vi "User Interface.vi"(8 "error in":errorcluster, 11 "Inset In":refnum<class "Inset.lvclass">) -> (0 "error out":errorcluster, 3 "Inset Out":refnum<class "Inset.lvclass">)   [LabVIEW 2019, in "Inset.lvclass"]
uses:
  Inset.lvclass
  BigMAQ/BigMAQ.lvclass
  Parse/ParseXML/Image.ctl
  Parse/ParseXML/ParseSVG.lvclass
  Parse/EditSVG/EditSVG.lvclass
  <vilib>/LabVIEW Open Source Project/OpenURI/openURI.lvlib
  <vilib>/LabVIEW Open Source Project/Data Manipulation/Scalar/OpenScalar.lvlib
panel:
  in  "Apply":bool
  in  "Cancel":bool
  out "SVG File":path caption="Path"
  in  "Inset Page":u32 caption="Numeric" max=3
  in  "Inset Data Range":cluster{sgl, sgl}(slide)={100.0, 0.0} scale=0.0..100.0
  in  "Inset Image":path caption="Path"
  in  "Background Page":u32 caption="Numeric" max=3
  in  "Background Data Range":cluster{sgl, sgl}(slide)={100.0, 0.0} scale=0.0..100.0
  out "Background Image":path caption="Path"
  in  "Inset Collapse":bool
  out "INST Render":T1(plugin-control)
  in  "Background Collapse":bool
  out "BGND Render":T1(plugin-control)
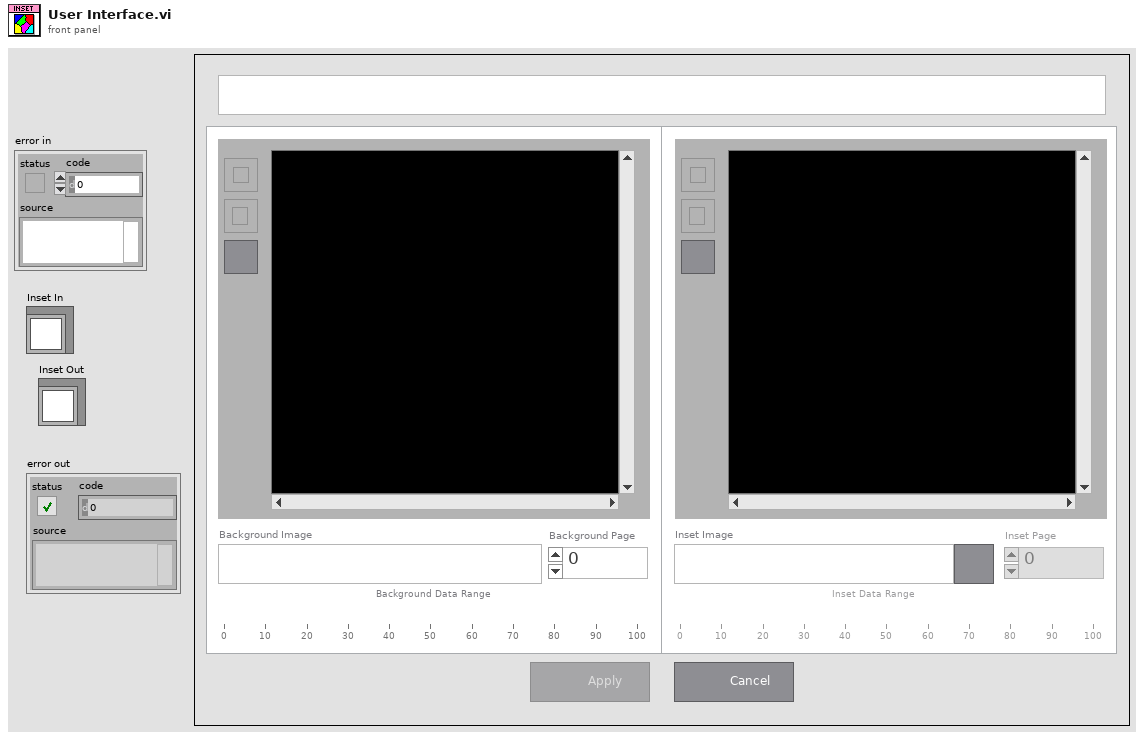
[diagram p1: front panel]
types:
  T1 = typedef "IMAQ Image.ctl" = refnum<image>
  T2 = enum32{"Invalid", "Standard", "Closed", "Hidden", "Minimized", "Maximized"}
  T3 = enum32{"invalid app kind", "Development System", "Run Time System", "Student Edition", "Embedded LabVIEW", "Evaluation", "Custom"}
  T4 = enum8{"Enabled", "Disabled", "Disabled and Grayed Out"}
  T5 = typedef "ParseSVG.lvclass/Image.ctl" = cluster{"x":string, "y":string, "width":string, "height":string, "xlink:href":string, "id":string, "transform":string}
  T6 = cluster{"Core":cluster{"Current VI Reference":refnum<vi>, "Close Panel on Exit?":bool}, "BGND Data":cluster{"YOffset":dbl, "XOffset":dbl, "ScanSize":dbl}, "INST Data":cluster{"YOffset":dbl, "XOffset":dbl, "ScanSize":dbl}, "SVG Image Data":T5, "Exists?":bool, "Existing id":string}
  T7 = cluster{"YOffset":dbl, "XOffset":dbl, "ScanSize":dbl}
  T8 = cluster{"Current VI Reference":refnum<vi>, "Close Panel on Exit?":bool}
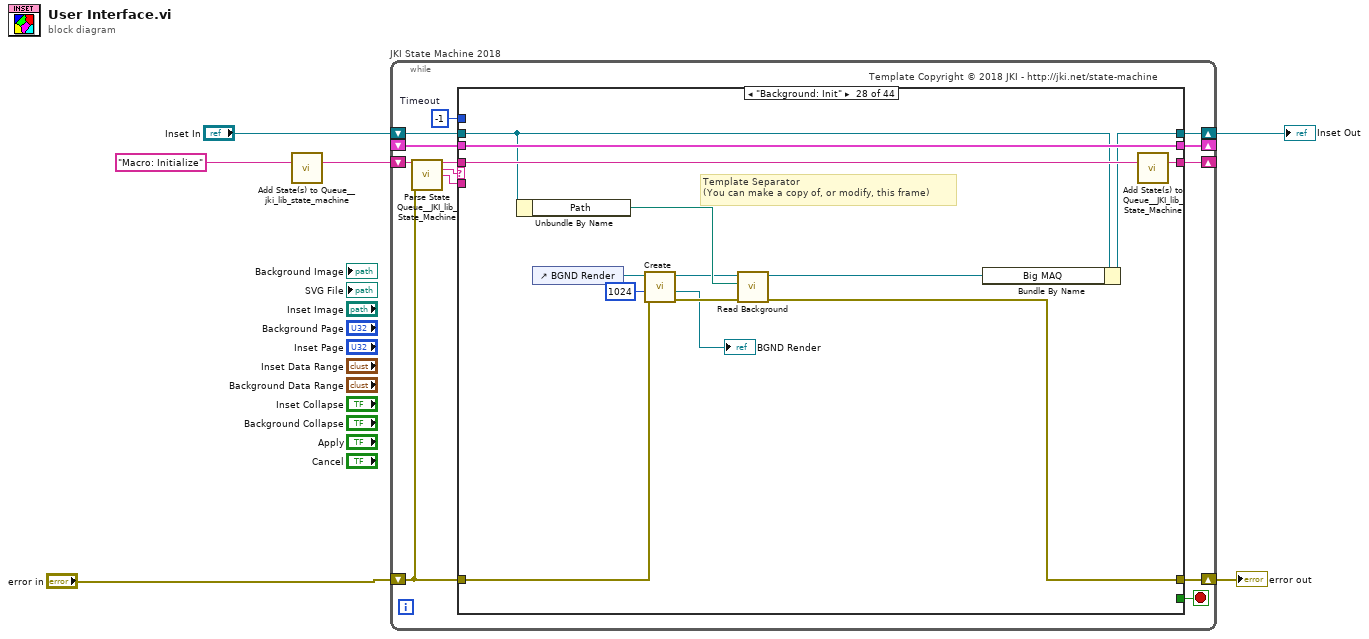
[diagram p0: block diagram]
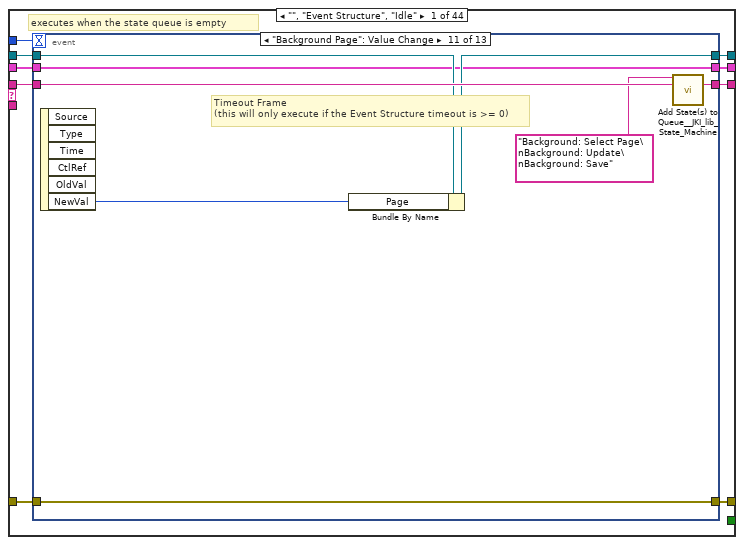
[diagram p2: hidden frame]
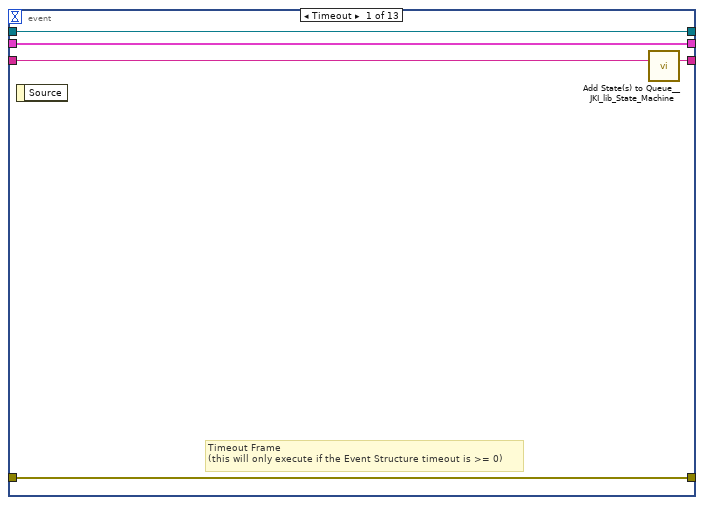
[diagram p3: hidden frame]
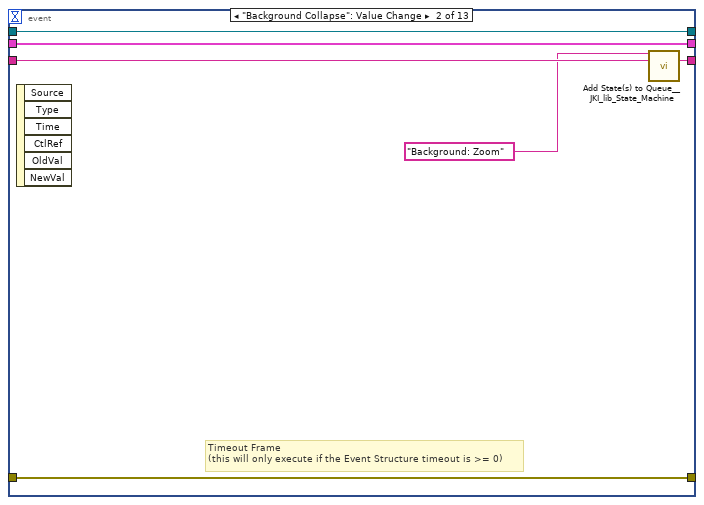
[diagram p4: hidden frame]
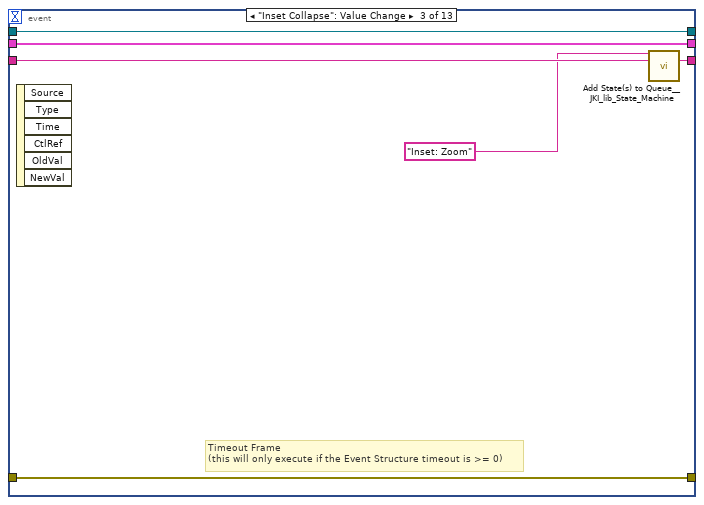
[diagram p5: hidden frame]
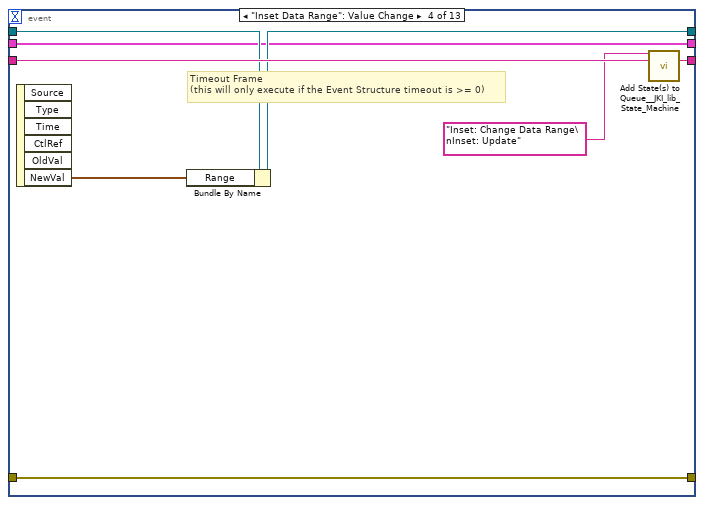
[diagram p6: hidden frame]
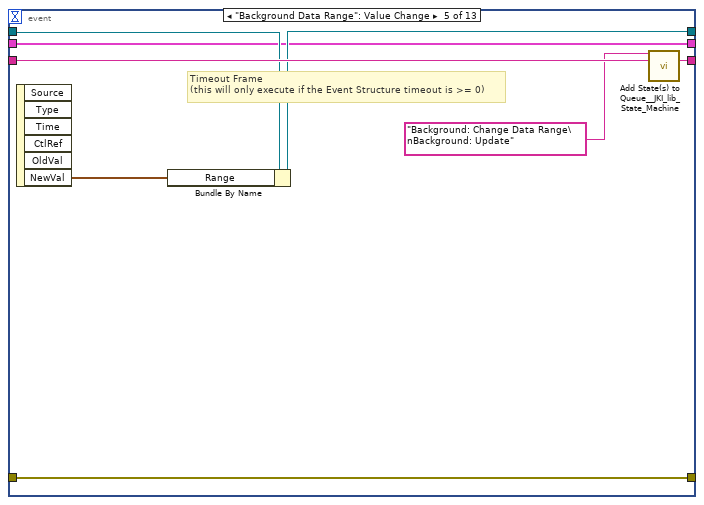
[diagram p7: hidden frame]
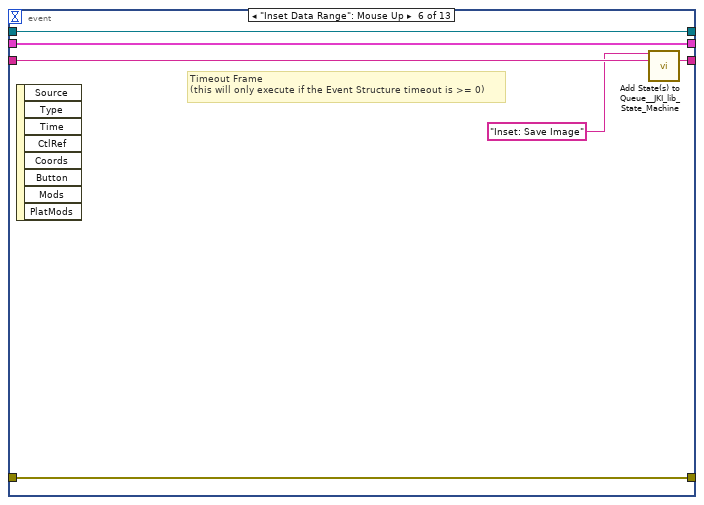
[diagram p8: hidden frame]
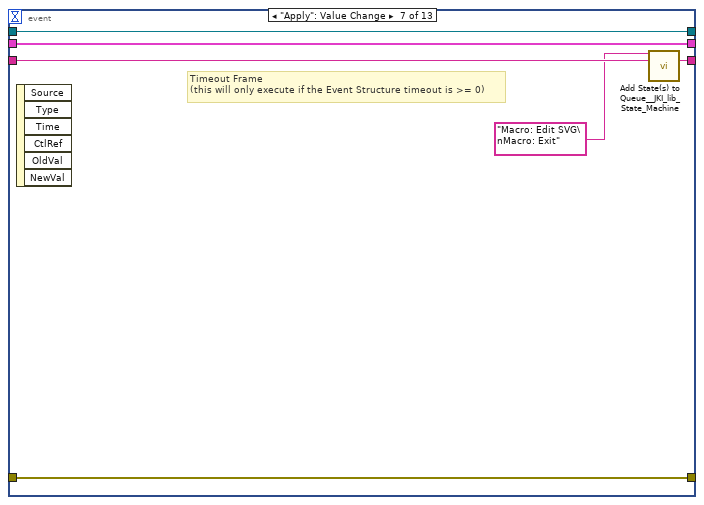
[diagram p9: hidden frame]
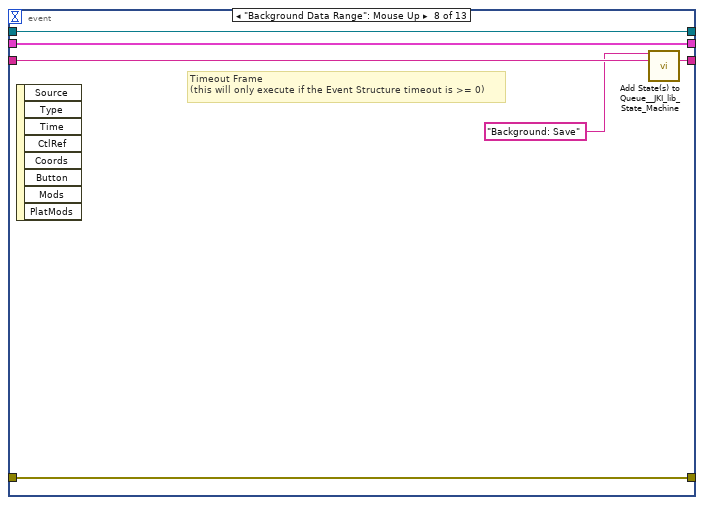
[diagram p10: hidden frame]
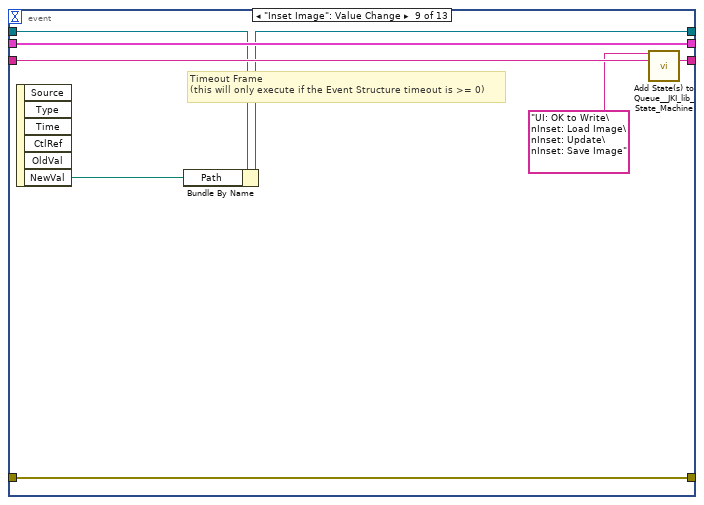
[diagram p11: hidden frame]
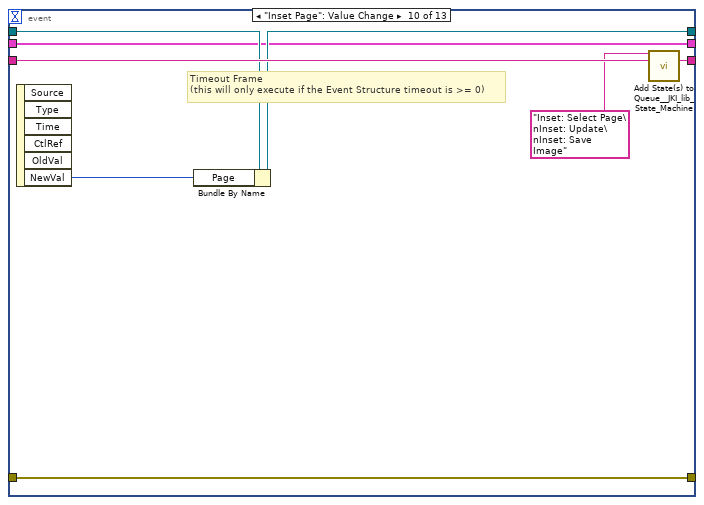
[diagram p12: hidden frame]
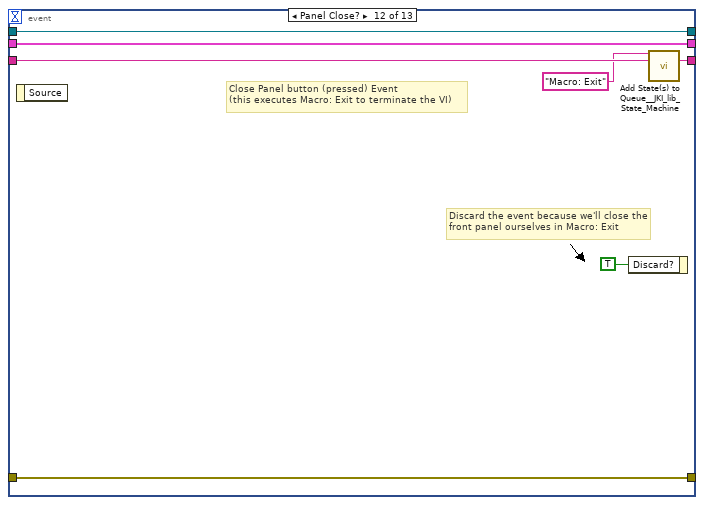
[diagram p13: hidden frame]
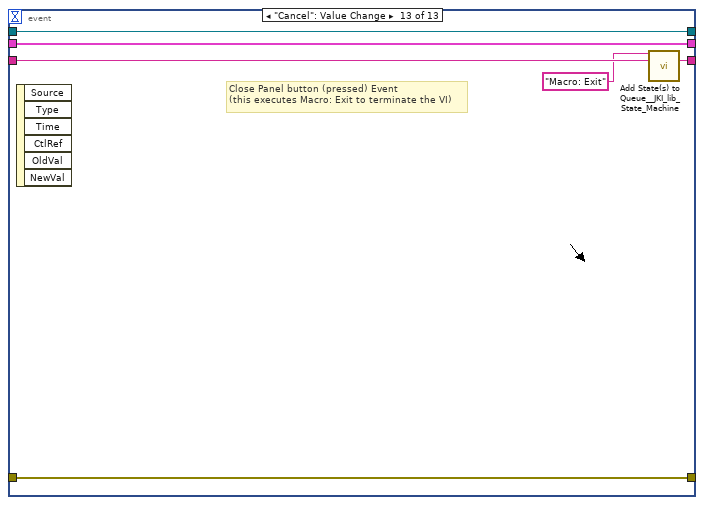
[diagram p14: hidden frame]
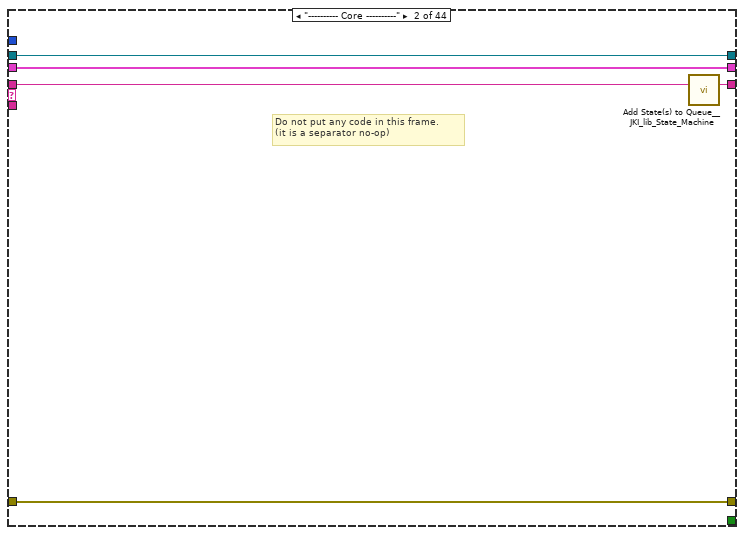
[diagram p15: hidden frame]
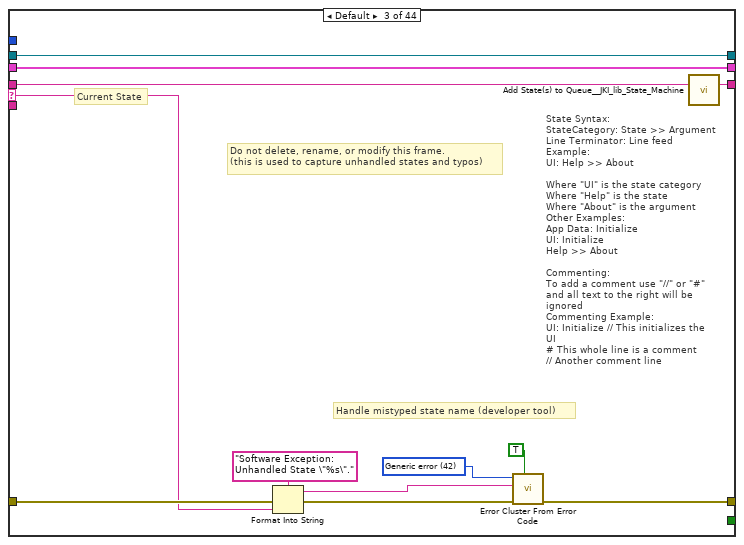
[diagram p16: hidden frame]
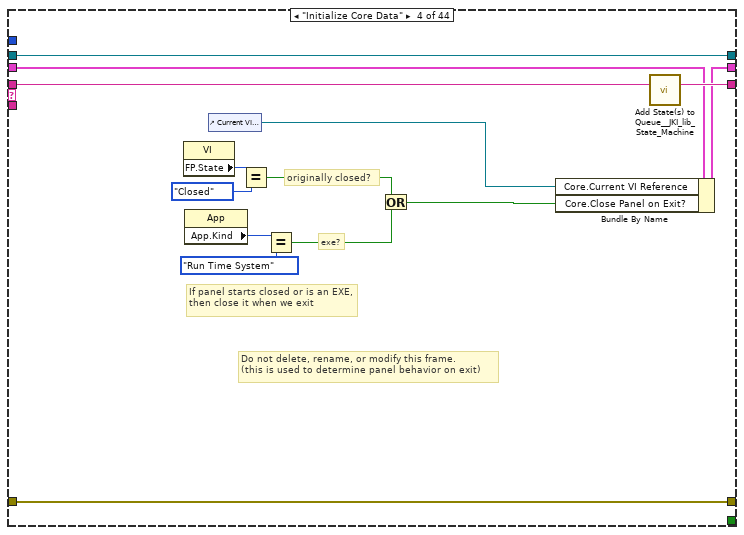
[diagram p17: hidden frame]
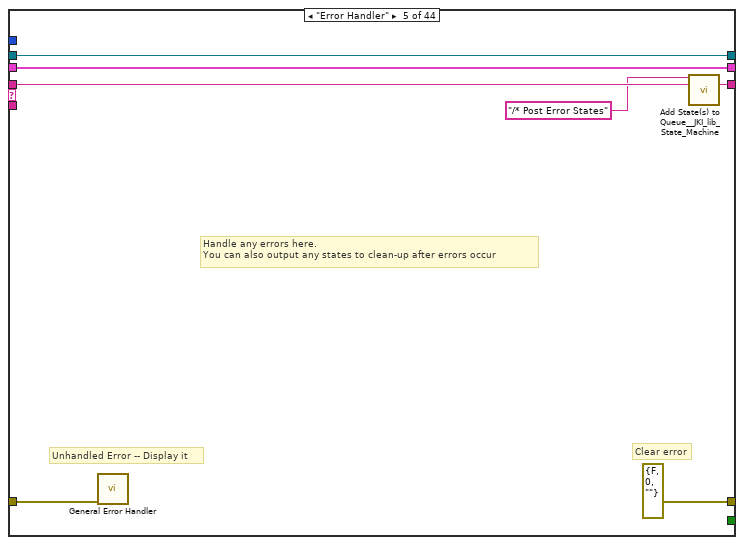
[diagram p18: hidden frame]
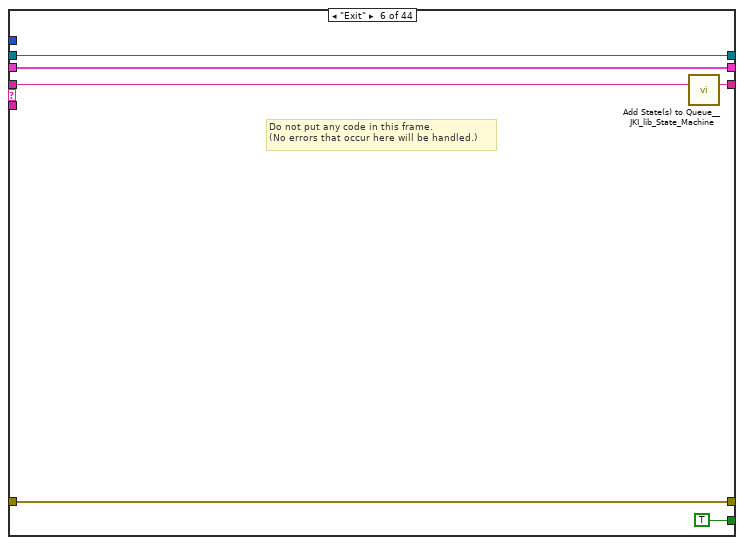
[diagram p19: hidden frame]
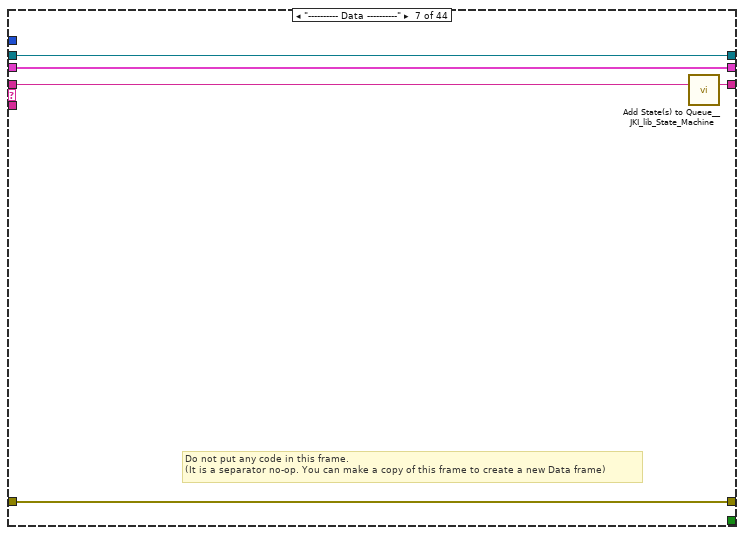
[diagram p20: hidden frame]
diagram:
  n1 = call <vilib>:"Add State(s) to Queue__jki_lib_state_machine.vi"("State(s) in (\"\")"="Macro: Initialize") -> ("States Out"=w6:string)  [unwired: 14 in]
  n2 = while "JKI State Machine 2018" {
    shift-right: [w12] -> _
    shift-left: _ -> [w11]
    shift-right: [w15] -> w4
    shift-left: "error in" -> [w9]
    shift-right: [w14] -> _
    shift-left: w6 -> [w16]
    shift-right: [w7] -> w1
    shift-left: "Inset In" -> [w8]
    stop <- w13 stop-if-true
    w10 = -1  # Timeout
    # "Template Copyright © 2018 JKI - http://jki.net/state-machine"
    n3 = call <vilib>:"Parse State Queue__JKI_lib_State_Machine.vi"("State Queue"=w16, "Error In (no error)"=w9) -> ("Remaining States"=w18:string, "Current State"=w19:string, "Arguments"=w17:string)  [unwired: 11 in]
    n4 = case shown="\"Background: Init\"" w19 {
      selector: w19 -> [_ _ w123 _ _ _ _ _ _ _ _ _ _ _ _ _ _ _ _ _ _ _ _ _ _ _ _ _ _ _ _ _ _ _ _ _ _ _ _ _ _ _ _ _]
      tunnel: w18 -> [w28 w121 w127 w147 w154 w160 w165 w176 w183 w188 w204 w219 w226 w238 w308 w314 w320 w331 w342 w347 w361 w383 w392 w404 w417 w442 w449 w463 w479 w493 w504 w515 w524 w533 w542 w549 w558 w567 w587 w598 w612 w624 w636 w645]
      tunnel: w17 -> [_ _ _ _ _ _ _ _ _ _ _ _ w221 w232 _ _ _ _ _ _ _ _ _ _ _ _ _ _ _ _ _ _ _ _ _ _ _ _ _ _ _ _ _ _]
      tunnel: w11 -> [w26 w118 w125 w140 w151 w158 w162 _ w178 w185 w202 w207 w224 w234 w305 w311 w317 w327 w339 w344 w349 w370 w385 w393 w405 w426 w446 w461 w477 w484 w498 w509 w520 w531 w536 w545 w556 w561 w584 w590 w599 w615 w629 w637]
      tunnel: [w25 w119 w129 w144 errorcluster {"status"=FALSE, "code"=0, "source"=""} ("error out") w157 w163 w173 w179 w186 w190 w209 w222 w235 w306 w312 w318 w329 w340 w345 w357 w381 w390 w396 w410 w440 w447 w452 w468 w486 w500 w513 w522 w526 w538 w547 w551 w563 w575 w594 w608 w620 w631 w641] -> w15
      tunnel: w9 -> [w24 w119 w128 w144 w150 w157 w163 w173 w180 w186 w196 w208 w223 w236 w306 w312 w318 w329 w340 w345 w354 w381 w390 w395 w409 w440 w447 w459 w475 w485 w499 w512 w521 w525 w537 w547 w550 w562 w583 w593 w607 w619 w630 w640]
      tunnel: [w27 w120 w126 w146 w153 w159 w164 w175 w182 w187 w203 w218 w225 w237 w307 w313 w319 w330 w341 w346 w360 w382 w391 w403 w416 w441 w448 w462 w478 w492 w503 w514 w523 w532 w541 w548 w557 w566 w586 w597 w611 w623 w635 w644] -> w14
      tunnel: [_ _ _ _ _ TRUE _ _ _ _ _ _ _ _ _ _ _ _ _ _ _ _ _ _ _ _ _ _ _ _ _ _ _ _ _ _ _ _ _ _ _ _ _ _] -> w13
      tunnel: [w23 w118 w125 w145 w151 w158 w162 w174 w178 w185 w202 w207 w224 w234 w305 w311 w317 w327 w339 w344 w349 w371 w385 w393 w405 w426 w446 w461 w476 w484 w498 w509 w520 w531 w536 w545 w556 w561 w585 w590 w599 w615 w629 w637] -> w12
      tunnel: w10 -> [w22 _ _ _ _ _ _ _ _ _ _ _ _ _ _ _ _ _ _ _ _ _ _ _ _ _ _ _ _ _ _ _ _ _ _ _ _ _ _ _ _ _ _ _]
      tunnel: w8 -> [w21 w117 w122 w134 w148 w155 w161 w171 w177 w184 w201 w217 w220 w231 w304 w309 w315 w321 w332 w343 w352 w376 w388 w394 w406 w424 w444 w456 w464 w482 w494 w505 w516 w529 w534 w543 w554 w559 w570 w591 w600 w613 w627 w638]
      tunnel: [w20 w117 w122 w134 w148 w155 w161 w171 w177 w184 w201 w217 w220 w231 w304 w309 w315 w321 w332 w343 w353 w377 w386 w394 w407 w425 w445 w460 w465 w483 w495 w506 w517 w530 w535 w544 w555 w560 w571 w592 w601 w614 w628 w639] -> w7
      frame "", "Event Structure", "Idle" {
        # "executes when the state queue is empty"
        n5 = event shown="[10] \"Background Page\": Value Change" {
          selector: _ -> [_ _ _ _ _ _ _ _ _ _ _ _ _]
          dyn-events: _ -> [_ _ _ _ _ _ _ _ _ _ _ _ _]
          timeout: w22 -> [_ _ _ _ _ _ _ _ _ _ _ _ _]
          tunnel: w28 -> [w33 w39 w45 w53 w61 w67 w73 w79 w87 w95 w103 w110 w116]
          tunnel: [w32 w38 w44 w52 w60 w66 w72 w78 w86 w94 w102 w109 w115] -> w27
          tunnel: w26 -> [w30 w36 w42 w46 w55 w63 w69 w75 w82 w88 w96 w107 w113]
          tunnel: [w31 w37 w43 w51 w59 w65 w71 w77 w85 w93 w101 w108 w114] -> w25
          tunnel: w24 -> [w31 w37 w43 w51 w59 w65 w71 w77 w85 w93 w101 w108 w114]
          tunnel: [w30 w36 w42 w46 w55 w63 w69 w75 w82 w88 w96 w107 w113] -> w23
          tunnel: w21 -> [w29 w35 w41 w47 w56 w62 w68 w74 w80 w89 w98 w104 w111]
          tunnel: [w29 w35 w41 w48 w57 w62 w68 w74 w81 w90 w99 w104 w111] -> w20
          event Timeout {
            # "Timeout Frame\n(this will only execute if the Event Structure timeout is >= 0)"
            n6 = event-data() -> ()  [unwired: 1 in, 1 out]
            n7 = call <vilib>:"Add State(s) to Queue__JKI_lib_State_Machine.vi"("State(s) in (\"\")"=w33) -> ("States Out"=w32:string)  [unwired: 14 in]
          }
          event "Background Collapse": Value Change {
            # "Timeout Frame\n(this will only execute if the Event Structure timeout is >= 0)"
            n8 = event-data() -> ()  [unwired: 1 in, 6 out]
            n9 = call <vilib>:"Add State(s) to Queue__JKI_lib_State_Machine.vi"("State(s) in Front (\"\")"="Background: Zoom", "State(s) in (\"\")"=w39) -> ("States Out"=w38:string)  [unwired: 13 in]
          }
          event "Inset Collapse": Value Change {
            # "Timeout Frame\n(this will only execute if the Event Structure timeout is >= 0)"
            n10 = event-data() -> ()  [unwired: 1 in, 6 out]
            n11 = call <vilib>:"Add State(s) to Queue__JKI_lib_State_Machine.vi"("State(s) in Front (\"\")"="Inset: Zoom", "State(s) in (\"\")"=w45) -> ("States Out"=w44:string)  [unwired: 13 in]
          }
          event "Inset Data Range": Value Change {
            # "Timeout Frame\n(this will only execute if the Event Structure timeout is >= 0)"
            n12 = event-data() -> ("NewVal"=w49:cluster{sgl, sgl})  [unwired: 1 in, 5 out]
            n13 = Bundle By Name(cluster=w47, "Range"=w49) -> (w48:refnum<class "Inset.lvclass">)
            n14 = call <vilib>:"Add State(s) to Queue__JKI_lib_State_Machine.vi"("State(s) in Front (\"\")"="Inset: Change Data Range\nInset: Update" ("State(s) in Front (\"\")"), "State(s) in (\"\")"=w53) -> ("States Out"=w52:string)  [unwired: 13 in]
          }
          event "Background Data Range": Value Change {
            # "Timeout Frame\n(this will only execute if the Event Structure timeout is >= 0)"
            n15 = event-data() -> ("NewVal"=w54:cluster{sgl, sgl})  [unwired: 1 in, 5 out]
            n16 = Bundle By Name(cluster=w56, "Range"=w54) -> (w57:refnum<class "Inset.lvclass">)
            n17 = call <vilib>:"Add State(s) to Queue__JKI_lib_State_Machine.vi"("State(s) in Front (\"\")"="Background: Change Data Range\nBackground: Update" ("State(s) in Front (\"\")"), "State(s) in (\"\")"=w61) -> ("States Out"=w60:string)  [unwired: 13 in]
          }
          event "Inset Data Range": Mouse Up {
            # "Timeout Frame\n(this will only execute if the Event Structure timeout is >= 0)"
            n18 = event-data() -> ()  [unwired: 1 in, 8 out]
            n19 = call <vilib>:"Add State(s) to Queue__JKI_lib_State_Machine.vi"("State(s) in Front (\"\")"="Inset: Save Image" ("State(s) in Front (\"\")"), "State(s) in (\"\")"=w67) -> ("States Out"=w66:string)  [unwired: 13 in]
          }
          event "Apply": Value Change {
            # "Timeout Frame\n(this will only execute if the Event Structure timeout is >= 0)"
            n20 = event-data() -> ()  [unwired: 1 in, 6 out]
            n21 = call <vilib>:"Add State(s) to Queue__JKI_lib_State_Machine.vi"("State(s) in Front (\"\")"="Macro: Edit SVG\nMacro: Exit" ("State(s) in Front (\"\")"), "State(s) in (\"\")"=w73) -> ("States Out"=w72:string)  [unwired: 13 in]
          }
          event "Background Data Range": Mouse Up {
            # "Timeout Frame\n(this will only execute if the Event Structure timeout is >= 0)"
            n22 = event-data() -> ()  [unwired: 1 in, 8 out]
            n23 = call <vilib>:"Add State(s) to Queue__JKI_lib_State_Machine.vi"("State(s) in Front (\"\")"="Background: Save" ("State(s) in Front (\"\")"), "State(s) in (\"\")"=w79) -> ("States Out"=w78:string)  [unwired: 13 in]
          }
          event "Inset Image": Value Change {
            # "Timeout Frame\n(this will only execute if the Event Structure timeout is >= 0)"
            n24 = event-data() -> ("NewVal"=w83:path)  [unwired: 1 in, 5 out]
            n25 = Bundle By Name(cluster=w80, "Path"=w83) -> (w81:refnum<class "Inset.lvclass">)
            n26 = call <vilib>:"Add State(s) to Queue__JKI_lib_State_Machine.vi"("State(s) in Front (\"\")"="UI: OK to Write\nInset: Load Image\nInset: Update\nInset: Save Image" ("State(s) in Front (\"\")"), "State(s) in (\"\")"=w87) -> ("States Out"=w86:string)  [unwired: 13 in]
          }
          event "Inset Page": Value Change {
            # "Timeout Frame\n(this will only execute if the Event Structure timeout is >= 0)"
            n27 = event-data() -> ("NewVal"=w91:u32)  [unwired: 1 in, 5 out]
            n28 = Bundle By Name(cluster=w89, "Page"=w91) -> (w90:refnum<class "Inset.lvclass">)
            n29 = call <vilib>:"Add State(s) to Queue__JKI_lib_State_Machine.vi"("State(s) in Front (\"\")"="Inset: Select Page\nInset: Update\nInset: Save Image" ("State(s) in Front (\"\")"), "State(s) in (\"\")"=w95) -> ("States Out"=w94:string)  [unwired: 13 in]
          }
          event "Background Page": Value Change {
            # "Timeout Frame\n(this will only execute if the Event Structure timeout is >= 0)"
            n30 = event-data() -> ("NewVal"=w97:u32)  [unwired: 1 in, 5 out]
            n31 = Bundle By Name(cluster=w98, "Page"=w97) -> (w99:refnum<class "Inset.lvclass">)
            n32 = call <vilib>:"Add State(s) to Queue__JKI_lib_State_Machine.vi"("State(s) in Front (\"\")"="Background: Select Page\nBackground: Update\nBackground: Save" ("State(s) in Front (\"\")"), "State(s) in (\"\")"=w103) -> ("States Out"=w102:string)  [unwired: 13 in]
          }
          event Panel Close? {
            # "Discard the event because we'll close the front panel ourselves in Macro: Exit"
            # "Close Panel button (pressed) Event\n(this executes Macro: Exit to terminate the VI)"
            n33 = event-data() -> ()  [unwired: 1 in, 1 out]
            n34 = event-data("Discard?"=TRUE) -> ()  [unwired: 1 in, 1 out]
            n35 = call <vilib>:"Add State(s) to Queue__JKI_lib_State_Machine.vi"("State(s) in Front (\"\")"="Macro: Exit", "State(s) in (\"\")"=w110) -> ("States Out"=w109:string)  [unwired: 13 in]
          }
          event "Cancel": Value Change {
            # "Close Panel button (pressed) Event\n(this executes Macro: Exit to terminate the VI)"
            n36 = event-data() -> ()  [unwired: 1 in, 6 out]
            n37 = call <vilib>:"Add State(s) to Queue__JKI_lib_State_Machine.vi"("State(s) in Front (\"\")"="Macro: Exit", "State(s) in (\"\")"=w116) -> ("States Out"=w115:string)  [unwired: 13 in]
          }
        }
      }
      frame "---------- Core ----------" {
        # "Do not put any code in this frame.\n(it is a separator no-op)"
        n38 = call <vilib>:"Add State(s) to Queue__JKI_lib_State_Machine.vi"("State(s) in (\"\")"=w121) -> ("States Out"=w120:string)  [unwired: 14 in]
      }
      frame Default {
        w132 = 42 items=["No error", "Argument error", "Memory is full", "Out of zone", "End of file", "File already open", "Generic file I/O error", "File not found", "File permission error", "Disk is full", "Duplicate path", "Too many files open", "System feature not enabled", "Resource file not found", "Cannot add resource", "Resource not found", "Image not found", "Image memory error", "Pen does not exist", "Config type invalid", "Config token not found", "Config parse error", "Config memory error", "Bad external code format", "Bad external code offset", "External code not present", "Null window", "Destroy window error", "Null menu", "Print aborted", "Bad print record", "Print driver error", "Windows error during printing", "Memory error during printing", "Print dialog error", "Generic print error", "Invalid device refnum", "Device not found", "Device parameter error", "Device unit error", "Cannot open device", "Device call aborted", "Generic error", "Cancelled by user", "Object ID too low", "Object ID too high", "Object not in heap", "Unknown heap", "Unknown object (invalid DefProc)", "Unknown object (DefProc not in table)", "Message out of range", "Invalid (null) method", "Unknown message", "Manager call not supported", "Bad address", "Network operation in progress", "Network operation timed out", "Connection is busy", "Network attribute not supported", "Network error", "Address in use", "System out of memory", "Connection aborted", "Connection refused", "Not connected", "Already connected", "Connection closed", "Initialization error (interapplication manager)", "Bad occurrence", "Wait on unbound occurrence handler", "Occurrence queue overflow", "Datalog type conflict", "Unused", "Unrecognized type (interapplication manager)", "Memory corrupt", "Failed to make temporary DLL", "Old CIN version", "Drag socket not found", "Failed to load drop-object", "Failed to register OLE object", "Failed to release OLE object", "Format specifier type mismatch", "Unknown format specifier", "Too few format specifiers", "Too many format specifiers", "Scan failed", "Newer CIN version", "Error converting to variant", "Runtime menu error", "Password tampered", "Variant attribute not found", "Incompatible variant data type", "Event data is not available", "Event Store is not present", "Occurrence is not found", "Event Queue is not created", "Event info is not available", "Refnum passed is NULL", "Error retrieving Class GUID", "Error retrieving CoClass GUID", "Error retrieving TypeLib GUID.", "Bad built application magic bytes.", "Specific driver is different from the specific driver associated with the Logical Name.", "There is no session opened to the class driver.", "Max Error", "MAX - Error with config objects", "MAX - Error loading configuration", "MAX - Group not supported"]
        # "State Syntax:\nStateCategory: State >> Argument\nLine Terminator: Line feed\nExample:\nUI: Help >> About\n\nWhere \"UI\" is the state category\nWhere \"Help\" is the state\nWhere \"About\" is the argument\nOther Examples:\nApp Data: Initialize\nUI: Initialize\nHelp >> About\n\nCommenting:\nTo add a comment use \"//\" or \"#\" and all text to the right will be ignored\nCommenting Example:\nUI: Initialize // This initializes the UI\n# This whole line is a comment\n// Another comment line"
        # "Current State"
        # "Do not delete, rename, or modify this frame.\n(this is used to capture unhandled states and typos)"
        # "Handle mistyped state name (developer tool)"
        n39 = Format Into String(format string="Software Exception: Unhandled State \"%s\"." ("message"), error in=w128, w123) -> (resulting string=w131:string, error out=w130:errorcluster)  [unwired: 1 in]
        n40 = call <vilib>:"Error Cluster From Error Code.vi"("show call chain? (False)"=TRUE, "error in (no error)"=w130, "error message (\"\")"=w131, "error code (0)"=w132) -> ("error out"=w129:errorcluster)  [unwired: 5 in]
        n41 = call <vilib>:"Add State(s) to Queue__JKI_lib_State_Machine.vi"("State(s) in (\"\")"=w127) -> ("States Out"=w126:string)  [unwired: 14 in]
      }
      frame "Initialize Core Data" {
        # "Do not delete, rename, or modify this frame.\n(this is used to determine panel behavior on exit)"
        # "originally closed?"
        # "exe?"
        # "If panel starts closed or is an EXE, then close it when we exit"
        n42 = property class="VI"() -> ("FP.State"=w137:T2)  [unwired: 2 in, 2 out]
        n43 = property class="App"() -> ("App.Kind"=w143:T3)  [unwired: 2 in, 2 out]
        n44 = control-ref of="Current VI Reference"() -> (w138:refnum<vi>)
        n45 = Equal?(x=w137, y=T2."Closed" ("Front Panel Window:State")) -> (x = y?=w135:bool)
        n46 = Equal?(x=w143, y=T3."Run Time System" ("Application:Kind")) -> (x = y?=w141:bool)
        n47 = Or(x=w135, y=w141) -> (x .or. y?=w139:bool)
        n48 = Bundle By Name(cluster=w140, "Core.Current VI Reference"=w138, "Core.Close Panel on Exit?"=w139) -> (w145:T6)
        n49 = call <vilib>:"Add State(s) to Queue__JKI_lib_State_Machine.vi"("State(s) in (\"\")"=w147) -> ("States Out"=w146:string)  [unwired: 14 in]
      }
      frame "Error Handler" {
        # "Unhandled Error -- Display it"
        # "Handle any errors here.\nYou can also output any states to clean-up after errors occur"
        # "Clear error"
        n50 = call <vilib>:"General Error Handler.vi"("error in (no error)"=w150) -> ()  [unwired: 10 in, 5 out]
        n51 = call <vilib>:"Add State(s) to Queue__JKI_lib_State_Machine.vi"("State(s) in Front (\"\")"="/* Post Error States", "State(s) in (\"\")"=w154) -> ("States Out"=w153:string)  [unwired: 13 in]
      }
      frame "Exit" {
        # "Do not put any code in this frame.\n(No errors that occur here will be handled.)"
        n52 = call <vilib>:"Add State(s) to Queue__JKI_lib_State_Machine.vi"("State(s) in (\"\")"=w160) -> ("States Out"=w159:string)  [unwired: 14 in]
      }
      frame "---------- Data ----------" {
        # "Do not put any code in this frame.\n(It is a separator no-op. You can make a copy of this frame to create a new Data frame)"
        n53 = call <vilib>:"Add State(s) to Queue__JKI_lib_State_Machine.vi"("State(s) in (\"\")"=w165) -> ("States Out"=w164:string)  [unwired: 14 in]
      }
      frame "Data: Initialize" {
        w166 = ""  # Existing id
        w167 = FALSE  # Exists?
        w168 = T5 {"x"="", "y"="", "width"="", "height"="", "xlink:href"="", "id"="", "transform"=""}  # SVG Image Data
        w169 = T7 {"YOffset"=0.0, "XOffset"=0.0, "ScanSize"=0.0}  # INST Data
        w170 = T7 {"YOffset"=0.0, "XOffset"=0.0, "ScanSize"=0.0}  # BGND Data
        w172 = T8 {"Current VI Reference"=refnum, "Close Panel on Exit?"=FALSE}  # Core
        # "do not delete - used by framework"
        # "Data names and types of shift register data are defined by this bundle."
        # "Initialize the shift-register data, here.\n(data names are defined by what you wire into the bundle function)"
        n54 = Bundle("Core"=w172, "BGND Data"=w170, "INST Data"=w169, "SVG Image Data"=w168, "Exists?"=w167, "Existing id"=w166) -> (w174:T6)  [unwired: 1 in]
        n55 = call <vilib>:"Add State(s) to Queue__JKI_lib_State_Machine.vi"("State(s) in (\"\")"=w176) -> ("States Out"=w175:string)  [unwired: 14 in]
      }
      frame "Data: Cleanup" {
        # "Cleanup any data and references, here.\n(this is called automatically, by the Macro: Exit)"
        n56 = Unbundle By Name(w178) -> ("Core.Current VI Reference"=w181:refnum<vi>)
        n57 = Close Reference(reference=w181, error in (no error)=w180) -> (error out=w179:errorcluster)
        n58 = call <vilib>:"Add State(s) to Queue__JKI_lib_State_Machine.vi"("State(s) in (\"\")"=w183) -> ("States Out"=w182:string)  [unwired: 14 in]
      }
      frame "---------- UI ----------" {
        # "Do not put any code in this frame.\n(It is a separator no-op. You can make a copy of this frame to create a new UI frame)"
        n59 = call <vilib>:"Add State(s) to Queue__JKI_lib_State_Machine.vi"("State(s) in (\"\")"=w188) -> ("States Out"=w187:string)  [unwired: 14 in]
      }
      frame "UI: OK to Write" {
        # "Do not put any code in this frame.\n(It is a separator no-op. You can make a copy of this frame to create a new UI frame)"
        n60 = Unbundle By Name(w201) -> ("Path"=w200:path)
        n61 = control-ref of="Apply"() -> (w189:refnum<vi>)
        n62 = Empty String/Path?(string/path=w200) -> (empty?=w199:bool)
        n63 = control-ref of="Inset Page"() -> (w194:refnum<vi>)
        n64 = control-ref of="Inset Data Range"() -> (w193:refnum<vi>)
        n65 = Select(t=T4."Disabled and Grayed Out" ("Disabled"), s=w199, f=T4."Enabled" ("Disabled")) -> (s? t:f=w191:T4)
        n66 = property class="Bool"(reference=w189, error in=w196, "DisabledEnum"=w191) -> (error out=w195:errorcluster)  [unwired: 1 out]
        n67 = property class="DigNum (strict)"(reference=w194, error in=w195, "DisabledEnum"=w191) -> (error out=w192:errorcluster)  [unwired: 1 out]
        n68 = property class="Slide (strict)"(reference=w193, error in=w192, "DisabledEnum"=w191) -> (error out=w190:errorcluster)  [unwired: 1 out]
        n69 = call <vilib>:"Add State(s) to Queue__JKI_lib_State_Machine.vi"("State(s) in (\"\")"=w204) -> ("States Out"=w203:string)  [unwired: 14 in]
      }
      frame "UI: Initialize" {
        # "Initialize the User Interface, here.\n(this is called automatically, by the Macro: Init)"
        n70 = Unbundle By Name(w207) -> ("Core.Current VI Reference"=w206:refnum<vi>)
        n71 = Unbundle By Name(w217) -> ("Path"=w216:path, "Range"=w211:cluster{sgl, sgl}, "Page"=w215:i32, "Path"=w214:path, "Range"=w212:cluster{sgl, sgl}, "Page"=w213:i32, "Path"=w210:path)
        n72 = local write "Background Image"(w216) -> ()
        n73 = local write "Background Page"(w215) -> ()
        n74 = local write "Inset Data Range"(w212) -> ()
        n75 = local write "SVG File"(w210) -> ()
        n76 = call <userlib>:"Fit VI window to Largest Dec__ogtk.vi"("error in (no error)"=w208, "border spacing (2 px)"=-4, "VI Ref (calling VI)"=w206) -> ("error out"=w209:errorcluster)  [unwired: 3 in, 1 out]
        n77 = local write "Background Data Range"(w211) -> ()
        n78 = local write "Inset Image"(w214) -> ()
        n79 = local write "Inset Page"(w213) -> ()
        n80 = call <vilib>:"Add State(s) to Queue__JKI_lib_State_Machine.vi"("State(s) in (\"\")"=w219) -> ("States Out"=w218:string)  [unwired: 14 in]
      }
      frame "UI: Cursor Set" {
        # "Argument"
        # "Set and Unset Cursor Busy.\n(Usage: \"UI: Cursor Set >> Busy|Idle\")"
        n81 = case shown="\"Idle\", Default" w221 {
          tunnel: w223 -> [w228 w230]
          tunnel: [w227 w229] -> w222
          frame "Idle", Default {
            n82 = call <vilib>:"Unset Busy.vi"("error in (no error)"=w228) -> ("error out"=w227:errorcluster)  [unwired: 10 in]
          }
          frame "Busy" {
            n83 = call <vilib>:"Set Busy.vi"("error in (no error)"=w230) -> ("error out"=w229:errorcluster)  [unwired: 9 in, 1 out]
          }
        }
        n84 = call <vilib>:"Add State(s) to Queue__JKI_lib_State_Machine.vi"("State(s) in (\"\")"=w226) -> ("States Out"=w225:string)  [unwired: 14 in]
      }
      frame "UI: Front Panel State" {
        # "Argument"
        # "Set Front Panel Open or Closed\n(Usage: \"UI: Front Panel State >> Open|Close\")"
        n85 = Unbundle By Name(w234) -> ("Core.Current VI Reference"=w233:refnum<vi>)
        n86 = case shown="\"Open\", \"Standard\", Default" w232 {
          tunnel: w236 -> [w244 w259 w270 w283 w296]
          tunnel: [w246 w260 w272 w285 w298] -> w235
          tunnel: w233 -> [w245 w257 w271 w284 w297]
          frame "Open", "Standard", Default {
            w239 = T2."Standard" ("State")
            n87 = property class="VI"(reference=w245, error in=w244) -> (reference out=w242:refnum<vi>, error out=w243:errorcluster, "FP.State"=w241:T2)
            n88 = Not Equal?(x=w241, y=w239) -> (x != y?=w240:bool)
            n89 = case shown="False" w240 {
              tunnel: [w250 w252] -> w246
              tunnel: w243 -> [w249 w252]
              tunnel: w242 -> [w248 _]
              tunnel: w239 -> [w247 _]
              frame True {
                n90 = invoke class="VI" method="FP.Open"(reference=w248, error in=w249, "Activate"=TRUE, "State"=w247) -> (error out=w250:errorcluster)  [unwired: 1 in, 4 out]
              }
              frame False {
              }
            }
          }
          frame "Close", "Closed" {
            n91 = property class="VI"(reference=w257, error in=w259) -> (reference out=w256:refnum<vi>, error out=w258:errorcluster, "FP.State"=w254:T2)
            n92 = Not Equal?(x=w254, y=T2."Closed" ("Front Panel Window:State")) -> (x != y?=w253:bool)
            n93 = case shown="True" w253 {
              tunnel: [w261 w264] -> w260
              tunnel: w258 -> [w261 w263]
              tunnel: w256 -> [_ w262]
              frame False {
              }
              frame True {
                n94 = invoke class="VI" method="FP.Close"(reference=w262, error in=w263) -> (error out=w264:errorcluster)  [unwired: 1 in, 2 out]
              }
            }
          }
          frame "Hidden", "Hide" {
            w265 = T2."Hidden" ("State")
            n95 = property class="VI"(reference=w271, error in=w270) -> (reference out=w268:refnum<vi>, error out=w269:errorcluster, "FP.State"=w267:T2)
            n96 = Not Equal?(x=w267, y=w265) -> (x != y?=w266:bool)
            n97 = case shown="True" w266 {
              tunnel: [w276 w277] -> w272
              tunnel: w269 -> [w275 w277]
              tunnel: w268 -> [w274 _]
              tunnel: w265 -> [w273 _]
              frame True {
                n98 = invoke class="VI" method="FP.Open"(reference=w274, error in=w275, "State"=w273) -> (error out=w276:errorcluster)  [unwired: 2 in, 4 out]
              }
              frame False {
              }
            }
          }
          frame "Minimize", "Minimized" {
            w278 = T2."Minimized" ("State")
            n99 = property class="VI"(reference=w284, error in=w283) -> (reference out=w281:refnum<vi>, error out=w282:errorcluster, "FP.State"=w280:T2)
            n100 = Not Equal?(x=w280, y=w278) -> (x != y?=w279:bool)
            n101 = case shown="True" w279 {
              tunnel: [w289 w290] -> w285
              tunnel: w282 -> [w288 w290]
              tunnel: w281 -> [w287 _]
              tunnel: w278 -> [w286 _]
              frame True {
                n102 = invoke class="VI" method="FP.Open"(reference=w287, error in=w288, "State"=w286) -> (error out=w289:errorcluster)  [unwired: 2 in, 4 out]
              }
              frame False {
              }
            }
          }
          frame "Maximize", "Maximized" {
            w291 = T2."Maximized" ("State")
            n103 = property class="VI"(reference=w297, error in=w296) -> (reference out=w294:refnum<vi>, error out=w295:errorcluster, "FP.State"=w293:T2)
            n104 = Not Equal?(x=w293, y=w291) -> (x != y?=w292:bool)
            n105 = case shown="True" w292 {
              tunnel: [w302 w303] -> w298
              tunnel: w295 -> [w301 w303]
              tunnel: w294 -> [w300 _]
              tunnel: w291 -> [w299 _]
              frame True {
                n106 = invoke class="VI" method="FP.Open"(reference=w300, error in=w301, "State"=w299) -> (error out=w302:errorcluster)  [unwired: 2 in, 4 out]
              }
              frame False {
              }
            }
          }
        }
        n107 = call <vilib>:"Add State(s) to Queue__JKI_lib_State_Machine.vi"("State(s) in (\"\")"=w238) -> ("States Out"=w237:string)  [unwired: 14 in]
      }
      frame "---------- Macro ----------" {
        # "Do not put any code in this frame.\n(It is a separator no-op. You can make a copy of this frame to create a new Macro frame)"
        n108 = call <vilib>:"Add State(s) to Queue__JKI_lib_State_Machine.vi"("State(s) in (\"\")"=w308) -> ("States Out"=w307:string)  [unwired: 14 in]
      }
      frame "Macro: Edit SVG" {
        # "Do not put any code in this frame.\n(It is a separator no-op. You can make a copy of this frame to create a new Macro frame)"
        n109 = call <vilib>:"Add State(s) to Queue__JKI_lib_State_Machine.vi"("State(s) in Front (\"\")"="SVG: Read\nSVG: Convert Data\nSVG: Inset href\nSVG: Generate ID\nSVG: Insert Inset\nSVG: Write", "State(s) in (\"\")"=w314) -> ("States Out"=w313:string)  [unwired: 13 in]
      }
      frame "Macro: Initialize Insert" {
        # "Do not put any code in this frame.\n(It is a separator no-op. You can make a copy of this frame to create a new Macro frame)"
        n110 = call <vilib>:"Add State(s) to Queue__JKI_lib_State_Machine.vi"("State(s) in Front (\"\")"="//Inset: Init UI\nInset: Load Image\nInset: Select Page\nInset: Change Data Range\nInset: Update\nInset: Save Image", "State(s) in (\"\")"=w320) -> ("States Out"=w319:string)  [unwired: 13 in]
      }
      frame "Macro: Initialize" {
        w328 = "Data: Initialize\nInitialize Core Data\nUI: Initialize\nUI: OK to Write\nUI: Front Panel State >> Open\nBackground: Init\n//Background: Update\nBackground: Select Page\nBackground: Change Data Range\nBackground: Get Data\nBackground: Update\nInset: Init UI"  # Data: Initialize Initialize Core Data UI: Initialize UI: OK to Write UI: Front Panel State >> Open Background: Init //Background: Update Background: Select Page Background: Change Data Range Background: Get Data Background: Update Inset: Init UI
        # "Initialization Macro\n(This is called once, when the VI starts)"
        n111 = Unbundle By Name(w321) -> ("Path"=w326:path)
        n112 = Empty String/Path?(string/path=w326) -> (empty?=w325:bool)
        n113 = Select(t="", s=w325, f="Macro: Initialize Insert") -> (s? t:f=w322:string)
        n114 = call <vilib>:"Add State(s) to Queue__JKI_lib_State_Machine.vi"("State(s) in Front (\"\")"=w328, "State(s) in (\"\")"=w331, "State(s) at Back (\"\")"=w322) -> ("States Out"=w330:string)  [unwired: 12 in]
      }
      frame "Macro: Exit" {
        # "Exit Macro\n(This is called once, when the VI exits)"
        n115 = Unbundle By Name(w339) -> ("Core.Close Panel on Exit?"=w338:bool)
        n116 = Select(t="UI: Front Panel State >> Close", s=w338, f="") -> (s? t:f=w335:string)
        n117 = call <vilib>:"Add State(s) to Queue__JKI_lib_State_Machine.vi"("State(s) in (\"\")"=w335, "State(s) at Back (\"\")"="Background: Cleanup\nInset: Cleanup\nData: Cleanup\nExit") -> ("States Out"=w333:string)  [unwired: 13 in]
        n118 = call <vilib>:"Add State(s) to Queue__JKI_lib_State_Machine.vi"("State(s) in Front (\"\")"=w333, "State(s) in (\"\")"=w342) -> ("States Out"=w341:string)  [unwired: 13 in]
      }
      frame "---------- SVG ----------" {
        # "Template Separator\n(You can make a copy of, or modify, this frame)"
        n119 = call <vilib>:"Add State(s) to Queue__JKI_lib_State_Machine.vi"("State(s) in (\"\")"=w347) -> ("States Out"=w346:string)  [unwired: 14 in]
      }
      frame "SVG: Insert Inset" {
        w359 = T5 {"x"="", "y"="", "width"="", "height"="", "xlink:href"="", "id"="", "transform"=""}  # image
        # "If the inset already exists, no need to add another below it... Just update image"
        # "Template Separator\n(You can make a copy of, or modify, this frame)"
        n120 = Unbundle By Name(w349) -> ("Exists?"=w348:bool)
        n121 = Unbundle By Name(w352) -> ("Image Data"=w356:T5, "XML"=w351:string, "id"=w355:string)
        n122 = Variant To Data(error in=w354, type=w359, Variant=w356) -> (data=w358:T5, error out=w357:errorcluster)
        n123 = case shown="False" w348 {
          tunnel: w358 -> [w365 _]
          tunnel: w355 -> [w364 _]
          tunnel: w351 -> [w363 w368]
          tunnel: [w362 w368] -> w350
          frame False {
            n124 = call "Place New Object After ID Object.vi"("Named Cluster"=w365, "Identifying Attribute Value"=w364, "Identifying Attribute Type"="id", "Element Type"="image", "XML String"=w363) -> ("Edited XML"=w362:string)  [unwired: 6 in]
          }
          frame True {
          }
        }
        n125 = Bundle By Name(cluster=w352, "XML"=w350) -> (w353:refnum<class "Inset.lvclass">)
        n126 = call <vilib>:"Add State(s) to Queue__JKI_lib_State_Machine.vi"("State(s) in (\"\")"=w361) -> ("States Out"=w360:string)  [unwired: 14 in]
      }
      frame "SVG: Inset href" {
        # "Template Separator\n(You can make a copy of, or modify, this frame)"
        n127 = Unbundle By Name(w376) -> ("Path"=w380:path, "Path"=w379:path, "XML"=w375:string)
        n128 = call "Get Inset Image JPG Name.vi"("Inset Data Path"=w379, "Inkscape Path"=w380) -> ("Inset JPG Name"=w378:string)  [unwired: 3 in]
        n129 = call <vilib>:"Percent-Encode String.vi"("String"=w378) -> ("Pct-Encoded String"=w372:string)  [unwired: 10 in]
        n130 = call "Search for Element by Attribute.vi"("Identifying Attribute Value"=w372, "Identifying Attribute Type"="xlink:href", "Element Type"="image", "XML String"=w375) -> ("Found?"=w369:bool)  [unwired: 4 in, 3 out]
        n131 = Bundle By Name(cluster=w376, "xlink:href"=w372) -> (w377:refnum<class "Inset.lvclass">)
        n132 = Bundle By Name(cluster=w370, "Exists?"=w369) -> (w371:T6)
        n133 = call <vilib>:"Add State(s) to Queue__JKI_lib_State_Machine.vi"("State(s) in (\"\")"=w383) -> ("States Out"=w382:string)  [unwired: 14 in]
      }
      frame "SVG: Generate ID" {
        # "I should find if there is an href to this image already."
        # "Template Separator\n(You can make a copy of, or modify, this frame)"
        n134 = Unbundle By Name(w388) -> ("XML"=w389:string)
        n135 = call "Generate Unique ID.vi"("Basename"="image", "XML String"=w389) -> ("Unique ID"=w387:string)  [unwired: 9 in]
        n136 = Bundle By Name(cluster=w388, "id"=w387, "id"=w387) -> (w386:refnum<class "Inset.lvclass">)
        n137 = call <vilib>:"Add State(s) to Queue__JKI_lib_State_Machine.vi"("State(s) in (\"\")"=w392) -> ("States Out"=w391:string)  [unwired: 14 in]
      }
      frame "SVG: Write" {
        # "Template Separator\n(You can make a copy of, or modify, this frame)"
        n138 = Unbundle By Name(w394) -> ("XML"=w397:string, "Path"=w398:path)
        n139 = Open/Create/Replace File(file path (use dialog)=w398, error in=w395) -> (refnum out=w400:refnum<file>, error out=w401:errorcluster)  [unwired: 4 in, 1 out]
        n140 = Write to Text File(file (use dialog)=w400, text=w397, error in=w401) -> (refnum out=w399:refnum<file>, error out=w402:errorcluster)  [unwired: 1 in, 1 out]
        n141 = Close File(refnum=w399, error in=w402) -> (error out=w396:errorcluster)  [unwired: 1 out]
        n142 = call <vilib>:"Add State(s) to Queue__JKI_lib_State_Machine.vi"("State(s) in (\"\")"=w404) -> ("States Out"=w403:string)  [unwired: 14 in]
      }
      frame "SVG: Read" {
        # "Template Separator\n(You can make a copy of, or modify, this frame)"
        n143 = Unbundle By Name(w406) -> ("Path"=w413:path)
        n144 = Open/Create/Replace File(file path (use dialog)=w413, error in=w409) -> (refnum out=w415:refnum<file>, error out=w411:errorcluster)  [unwired: 4 in, 1 out]
        n145 = Read from Text File(file (use dialog)=w415, error in=w411) -> (refnum out=w414:refnum<file>, text=w408:string, error out=w412:errorcluster)  [unwired: 2 in, 1 out]
        n146 = Close File(refnum=w414, error in=w412) -> (error out=w410:errorcluster)  [unwired: 1 out]
        n147 = Bundle By Name(cluster=w406, "XML"=w408) -> (w407:refnum<class "Inset.lvclass">)
        n148 = call <vilib>:"Add State(s) to Queue__JKI_lib_State_Machine.vi"("State(s) in (\"\")"=w417) -> ("States Out"=w416:string)  [unwired: 14 in]
      }
      frame "SVG: Convert Data" {
        # "Template Separator\n(You can make a copy of, or modify, this frame)"
        n149 = Unbundle By Name(w426) -> ("BGND Data.ScanSize"=w439:dbl, "BGND Data.XOffset"=w437:dbl, "BGND Data.YOffset"=w427:dbl, "INST Data.ScanSize"=w420:dbl, "INST Data.XOffset"=w435:dbl, "INST Data.YOffset"=w431:dbl)
        n150 = Divide(x=w439, y=2.0) -> (x/y=w433:dbl)
        n151 = Divide(x=w420, y=2.0) -> (x/y=w432:dbl)
        n152 = Add(x=w433, y=w427) -> (x+y=w428:dbl)
        n153 = Add(x=w432, y=w431) -> (x+y=w429:dbl)
        n154 = Subtract(x=w433, y=w437) -> (x-y=w434:dbl)
        n155 = Subtract(x=w432, y=w435) -> (x-y=w430:dbl)
        n156 = Subtract(x=w434, y=w430) -> (x-y=w423:dbl)
        n157 = Subtract(x=w428, y=w429) -> (x-y=w418:dbl)
        n158 = call <vilib>:"DoubleFloat (Scalar) to String.vi"("Value (Double)"=w423) -> ("Value (String)"=w422:string)  [unwired: 10 in]
        n159 = call <vilib>:"DoubleFloat (Scalar) to String.vi"("Value (Double)"=w418) -> ("Value (String)"=w421:string)  [unwired: 10 in]
        n160 = call <vilib>:"DoubleFloat (Scalar) to String.vi"("Value (Double)"=w420) -> ("Value (String)"=w419:string)  [unwired: 10 in]
        n161 = Bundle By Name(cluster=w424, "width"=w419, "height"=w419, "x"=w422, "y"=w421) -> (w425:refnum<class "Inset.lvclass">)
        n162 = call <vilib>:"Add State(s) to Queue__JKI_lib_State_Machine.vi"("State(s) in (\"\")"=w442) -> ("States Out"=w441:string)  [unwired: 14 in]
      }
      frame "---------- Background ----------" {
        # "Template Separator\n(You can make a copy of, or modify, this frame)"
        n163 = Unbundle By Name(w444) -> ("Big MAQ"=w443:refnum<class "BigMAQ.lvclass">)
        n164 = Bundle By Name(cluster=w444, "Big MAQ"=w443) -> (w445:refnum<class "Inset.lvclass">)
        n165 = call <vilib>:"Add State(s) to Queue__JKI_lib_State_Machine.vi"("State(s) in (\"\")"=w449) -> ("States Out"=w448:string)  [unwired: 14 in]
      }
      frame "Background: Init" {
        # "Template Separator\n(You can make a copy of, or modify, this frame)"
        n166 = Unbundle By Name(w456) -> ("Path"=w455:path)
        n167 = control-ref of="BGND Render"() -> (w458:refnum<vi>)
        n168 = call "Create.vi"("error in (no error)"=w459, "Resolution"=1024, "Reference"=w458) -> ("error out"=w453:errorcluster, "To Control"=→"BGND Render":T1, "BigMAQ out"=w454:refnum<class "BigMAQ.lvclass">)  [unwired: 6 in]
        n169 = call "Read Background.vi"("error in (no error)"=w453, "Path"=w455, "BigMAQ in"=w454) -> ("error out"=w452:errorcluster, "BigMAQ out"=w451:refnum<class "BigMAQ.lvclass">)  [unwired: 6 in, 1 out]
        n170 = Bundle By Name(cluster=w456, "Big MAQ"=w451) -> (w460:refnum<class "Inset.lvclass">)
        n171 = call <vilib>:"Add State(s) to Queue__JKI_lib_State_Machine.vi"("State(s) in (\"\")"=w463) -> ("States Out"=w462:string)  [unwired: 14 in]
      }
      frame "Background: Get Data" {
        # "This is already achieved for the inset upon loading the file. Since the file is already loaded here, we need to just look at the metadata"
        n172 = Unbundle By Name(w464) -> ("Big MAQ"=w467:refnum<class "BigMAQ.lvclass">)
        n173 = call-dynamic "Read Image Metadata.vi"("error in (no error)"=w475, "BigMAQ in"=w467) -> ("error out"=w469:errorcluster, "Image Metadata"=w474:variant, "BigMAQ out"=w472:refnum<class "BigMAQ.lvclass">)  [unwired: 7 in]
        n174 = call "Retrieve and Convert Data.vi"("error in (no error)"=w469, "Variant In"=w474) -> ("error out"=w470:errorcluster, "Info"=w471:T7, "Variant Out"=w473:variant)  [unwired: 7 in]
        n175 = Bundle By Name(cluster=w477, "BGND Data"=w471) -> (w476:T6)
        n176 = call-dynamic "Write Image Metadata.vi"("error in (no error)"=w470, "Image Metadata"=w473, "BigMAQ in"=w472) -> ("error out"=w468:errorcluster, "BigMAQ out"=w466:refnum<class "BigMAQ.lvclass">)  [unwired: 7 in]
        n177 = Bundle By Name(cluster=w464, "Big MAQ"=w466) -> (w465:refnum<class "Inset.lvclass">)
        n178 = call <vilib>:"Add State(s) to Queue__JKI_lib_State_Machine.vi"("State(s) in (\"\")"=w479) -> ("States Out"=w478:string)  [unwired: 14 in]
      }
      frame "Background: Change Data Range" {
        # "Template Separator\n(You can make a copy of, or modify, this frame)"
        n179 = Unbundle By Name(w482) -> ("Big MAQ"=w480:refnum<class "BigMAQ.lvclass">, "Range"=w491:cluster{sgl, sgl})
        n180 = Unbundle(w491) -> (w490:sgl, w489:sgl)
        n181 = Max & Min(x=w490, y=w489) -> (max(x,y)=w487:sgl, min(x,y)=w488:sgl)
        n182 = call "Change Data Range.vi"("error in"=w485, "Minimum"=w488, "Maximum"=w487, "BigMAQ in"=w480) -> ("error out"=w486:errorcluster, "BigMAQ out"=w481:refnum<class "BigMAQ.lvclass">)  [unwired: 6 in]
        n183 = Bundle By Name(cluster=w482, "Big MAQ"=w481) -> (w483:refnum<class "Inset.lvclass">)
        n184 = call <vilib>:"Add State(s) to Queue__JKI_lib_State_Machine.vi"("State(s) in (\"\")"=w493) -> ("States Out"=w492:string)  [unwired: 14 in]
      }
      frame "Background: Select Page" {
        # "Template Separator\n(You can make a copy of, or modify, this frame)"
        n185 = Unbundle By Name(w494) -> ("Big MAQ"=w496:refnum<class "BigMAQ.lvclass">, "Page"=w502:i32)
        n186 = call "Select Page.vi"("error in (no error)"=w499, "Page"=w502, "BigMAQ in"=w496) -> ("error out"=w500:errorcluster, "Corrected Page"=w501:u32, "BigMAQ out"=w497:refnum<class "BigMAQ.lvclass">)  [unwired: 6 in]
        n187 = Bundle By Name(cluster=w494, "Big MAQ"=w497, "Page"=w501) -> (w495:refnum<class "Inset.lvclass">)
        n188 = call <vilib>:"Add State(s) to Queue__JKI_lib_State_Machine.vi"("State(s) in (\"\")"=w504) -> ("States Out"=w503:string)  [unwired: 14 in]
      }
      frame "Background: Save" {
        # "Template Separator\n(You can make a copy of, or modify, this frame)"
        n189 = Unbundle By Name(w505) -> ("Big MAQ"=w508:refnum<class "BigMAQ.lvclass">, "Path"=w511:path)
        n190 = call "Get Background Image JPG Path.vi"("Inkscape Path"=w511) -> ("Background JPG Path"=w510:path)  [unwired: 2 in]
        n191 = call "Save Background.vi"("error in"=w512, "File Path"=w510, "BigMAQ in"=w508) -> ("error out"=w513:errorcluster, "BigMAQ out"=w507:refnum<class "BigMAQ.lvclass">)  [unwired: 7 in]
        n192 = Bundle By Name(cluster=w505, "Big MAQ"=w507) -> (w506:refnum<class "Inset.lvclass">)
        n193 = call <vilib>:"Add State(s) to Queue__JKI_lib_State_Machine.vi"("State(s) in (\"\")"=w515) -> ("States Out"=w514:string)  [unwired: 14 in]
      }
      frame "Background: Update" {
        # "Template Separator\n(You can make a copy of, or modify, this frame)"
        n194 = Unbundle By Name(w516) -> ("Big MAQ"=w519:refnum<class "BigMAQ.lvclass">)
        n195 = call "Update Control.vi"("error in"=w521, "BigMAQ in"=w519) -> ("error out"=w522:errorcluster, "BigMAQ out"=w518:refnum<class "BigMAQ.lvclass">)  [unwired: 8 in]
        n196 = Bundle By Name(cluster=w516, "Big MAQ"=w518) -> (w517:refnum<class "Inset.lvclass">)
        n197 = call <vilib>:"Add State(s) to Queue__JKI_lib_State_Machine.vi"("State(s) in (\"\")"=w524) -> ("States Out"=w523:string)  [unwired: 14 in]
      }
      frame "Background: Zoom" {
        # "Template Separator\n(You can make a copy of, or modify, this frame)"
        n198 = Unbundle By Name(w529) -> ("Big MAQ"=w528:refnum<class "BigMAQ.lvclass">)
        n199 = call "Zoom to Fit.vi"("error in"=w525, "BigMAQ in"=w528) -> ("error out"=w526:errorcluster, "BigMAQ out"=w527:refnum<class "BigMAQ.lvclass">)  [unwired: 7 in, 1 out]
        n200 = Bundle By Name(cluster=w529, "Big MAQ"=w527) -> (w530:refnum<class "Inset.lvclass">)
        n201 = call <vilib>:"Add State(s) to Queue__JKI_lib_State_Machine.vi"("State(s) in (\"\")"=w533) -> ("States Out"=w532:string)  [unwired: 14 in]
      }
      frame "Background: Cleanup" {
        # "Template Separator\n(You can make a copy of, or modify, this frame)"
        n202 = Unbundle By Name(w534) -> ("Big MAQ"=w540:refnum<class "BigMAQ.lvclass">)
        n203 = call "Destroy.vi"("error in"=w537, "BigMAQ in"=w540) -> ("error out"=w538:errorcluster, "BigMAQ out"=w539:refnum<class "BigMAQ.lvclass">)  [unwired: 8 in]
        n204 = Bundle By Name(cluster=w534, "Big MAQ"=w539) -> (w535:refnum<class "Inset.lvclass">)
        n205 = call <vilib>:"Add State(s) to Queue__JKI_lib_State_Machine.vi"("State(s) in (\"\")"=w542) -> ("States Out"=w541:string)  [unwired: 14 in]
      }
      frame "---------- Inset ----------" {
        # "Template Separator\n(You can make a copy of, or modify, this frame)"
        n206 = Unbundle By Name(w543) -> ("Big MAQ"=w546:refnum<class "BigMAQ.lvclass">)
        n207 = Bundle By Name(cluster=w543, "Big MAQ"=w546) -> (w544:refnum<class "Inset.lvclass">)
        n208 = call <vilib>:"Add State(s) to Queue__JKI_lib_State_Machine.vi"("State(s) in (\"\")"=w549) -> ("States Out"=w548:string)  [unwired: 14 in]
      }
      frame "Inset: Zoom" {
        # "Template Separator\n(You can make a copy of, or modify, this frame)"
        n209 = Unbundle By Name(w554) -> ("Big MAQ"=w553:refnum<class "BigMAQ.lvclass">)
        n210 = call "Zoom to Fit.vi"("error in"=w550, "BigMAQ in"=w553) -> ("error out"=w551:errorcluster, "BigMAQ out"=w552:refnum<class "BigMAQ.lvclass">)  [unwired: 7 in, 1 out]
        n211 = Bundle By Name(cluster=w554, "Big MAQ"=w552) -> (w555:refnum<class "Inset.lvclass">)
        n212 = call <vilib>:"Add State(s) to Queue__JKI_lib_State_Machine.vi"("State(s) in (\"\")"=w558) -> ("States Out"=w557:string)  [unwired: 14 in]
      }
      frame "Inset: Cleanup" {
        # "Template Separator\n(You can make a copy of, or modify, this frame)"
        n213 = Unbundle By Name(w559) -> ("Big MAQ"=w565:refnum<class "BigMAQ.lvclass">)
        n214 = call "Destroy.vi"("error in"=w562, "BigMAQ in"=w565) -> ("error out"=w563:errorcluster, "BigMAQ out"=w564:refnum<class "BigMAQ.lvclass">)  [unwired: 8 in]
        n215 = Bundle By Name(cluster=w559, "Big MAQ"=w564) -> (w560:refnum<class "Inset.lvclass">)
        n216 = call <vilib>:"Add State(s) to Queue__JKI_lib_State_Machine.vi"("State(s) in (\"\")"=w567) -> ("States Out"=w566:string)  [unwired: 14 in]
      }
      frame "Inset: Load Image" {
        # "Template Separator\n(You can make a copy of, or modify, this frame)"
        n217 = Unbundle By Name(w570) -> ("Big MAQ"=w573:refnum<class "BigMAQ.lvclass">, "Path"=w572:path)
        n218 = call "Read Background.vi"("error in (no error)"=w583, "Path"=w572, "BigMAQ in"=w573) -> ("error out"=w574:errorcluster, "BigMAQ out"=w577:refnum<class "BigMAQ.lvclass">)  [unwired: 6 in, 1 out]
        n219 = call-dynamic "Read Image Metadata.vi"("error in (no error)"=w574, "BigMAQ in"=w577) -> ("error out"=w578:errorcluster, "Image Metadata"=w582:variant, "BigMAQ out"=w580:refnum<class "BigMAQ.lvclass">)  [unwired: 7 in]
        n220 = call "Retrieve and Convert Data.vi"("error in (no error)"=w578, "Variant In"=w582) -> ("error out"=w579:errorcluster, "Info"=w576:T7, "Variant Out"=w581:variant)  [unwired: 7 in]
        n221 = call-dynamic "Write Image Metadata.vi"("error in (no error)"=w579, "Image Metadata"=w581, "BigMAQ in"=w580) -> ("error out"=w575:errorcluster, "BigMAQ out"=w569:refnum<class "BigMAQ.lvclass">)  [unwired: 7 in]
        n222 = Bundle By Name(cluster=w570, "Big MAQ"=w569) -> (w571:refnum<class "Inset.lvclass">)
        n223 = Bundle By Name(cluster=w584, "INST Data"=w576) -> (w585:T6)
        n224 = call <vilib>:"Add State(s) to Queue__JKI_lib_State_Machine.vi"("State(s) in Front (\"\")"="Inset: Select Page" ("State(s) in Front (\"\")"), "State(s) in (\"\")"=w587) -> ("States Out"=w586:string)  [unwired: 13 in]
      }
      frame "Inset: Select Page" {
        # "Template Separator\n(You can make a copy of, or modify, this frame)"
        n225 = Unbundle By Name(w591) -> ("Big MAQ"=w596:refnum<class "BigMAQ.lvclass">, "Page"=w589:i32)
        n226 = call "Select Page.vi"("error in (no error)"=w593, "Page"=w589, "BigMAQ in"=w596) -> ("error out"=w594:errorcluster, "Corrected Page"=w588:u32, "BigMAQ out"=w595:refnum<class "BigMAQ.lvclass">)  [unwired: 6 in]
        n227 = Bundle By Name(cluster=w591, "Big MAQ"=w595, "Page"=w588) -> (w592:refnum<class "Inset.lvclass">)
        n228 = local write "Inset Page"(w588) -> ()
        n229 = call <vilib>:"Add State(s) to Queue__JKI_lib_State_Machine.vi"("State(s) in (\"\")"=w598) -> ("States Out"=w597:string)  [unwired: 14 in]
      }
      frame "Inset: Change Data Range" {
        # "Template Separator\n(You can make a copy of, or modify, this frame)"
        n230 = Unbundle By Name(w600) -> ("Big MAQ"=w610:refnum<class "BigMAQ.lvclass">, "Range"=w606:cluster{sgl, sgl})
        n231 = Unbundle(w606) -> (w605:sgl, w604:sgl)
        n232 = Max & Min(x=w605, y=w604) -> (max(x,y)=w603:sgl, min(x,y)=w602:sgl)
        n233 = call "Change Data Range.vi"("error in"=w607, "Minimum"=w602, "Maximum"=w603, "BigMAQ in"=w610) -> ("error out"=w608:errorcluster, "BigMAQ out"=w609:refnum<class "BigMAQ.lvclass">)  [unwired: 6 in]
        n234 = Bundle By Name(cluster=w600, "Big MAQ"=w609) -> (w601:refnum<class "Inset.lvclass">)
        n235 = call <vilib>:"Add State(s) to Queue__JKI_lib_State_Machine.vi"("State(s) in (\"\")"=w612) -> ("States Out"=w611:string)  [unwired: 14 in]
      }
      frame "Inset: Save Image" {
        # "Template Separator\n(You can make a copy of, or modify, this frame)"
        n236 = Unbundle By Name(w613) -> ("Big MAQ"=w621:refnum<class "BigMAQ.lvclass">, "Path"=w618:path, "Path"=w617:path)
        n237 = call "Get Inset Image JPG Path.vi"("Inset Data Path"=w617, "Inkscape Path"=w618) -> ("Inset JPG Path"=w616:path)  [unwired: 3 in]
        n238 = call "Save Background.vi"("error in"=w619, "File Path"=w616, "BigMAQ in"=w621) -> ("error out"=w620:errorcluster, "BigMAQ out"=w622:refnum<class "BigMAQ.lvclass">)  [unwired: 7 in]
        n239 = Bundle By Name(cluster=w613, "Big MAQ"=w622) -> (w614:refnum<class "Inset.lvclass">)
        n240 = call <vilib>:"Add State(s) to Queue__JKI_lib_State_Machine.vi"("State(s) in (\"\")"=w624) -> ("States Out"=w623:string)  [unwired: 14 in]
      }
      frame "Inset: Init UI" {
        # "Template Separator\n(You can make a copy of, or modify, this frame)"
        n241 = control-ref of="INST Render"() -> (w633:refnum<vi>)
        n242 = call "Create.vi"("error in (no error)"=w630, "Resolution"=1024, "Reference"=w633) -> ("error out"=w631:errorcluster, "To Control"=w626:T1, "BigMAQ out"=w634:refnum<class "BigMAQ.lvclass">)  [unwired: 6 in]
        "INST Render" <- w626
        n243 = Type Cast(type=u8[] [], x=w626) -> ()  [unwired: 1 out]
        n244 = Bundle By Name(cluster=w627, "Big MAQ"=w634) -> (w628:refnum<class "Inset.lvclass">)
        n245 = call <vilib>:"Add State(s) to Queue__JKI_lib_State_Machine.vi"("State(s) in (\"\")"=w636) -> ("States Out"=w635:string)  [unwired: 14 in]
      }
      frame "Inset: Update" {
        # "Template Separator\n(You can make a copy of, or modify, this frame)"
        n246 = Unbundle By Name(w638) -> ("Big MAQ"=w643:refnum<class "BigMAQ.lvclass">)
        n247 = call "Update Control.vi"("error in"=w640, "BigMAQ in"=w643) -> ("error out"=w641:errorcluster, "BigMAQ out"=w642:refnum<class "BigMAQ.lvclass">)  [unwired: 8 in]
        n248 = Bundle By Name(cluster=w638, "Big MAQ"=w642) -> (w639:refnum<class "Inset.lvclass">)
        n249 = call <vilib>:"Add State(s) to Queue__JKI_lib_State_Machine.vi"("State(s) in (\"\")"=w645) -> ("States Out"=w644:string)  [unwired: 14 in]
      }
    }
  }
  "error out" <- w4
  "Inset Out" <- w1
